vi "Get Moving Status.vi"(8 "error in (no error)":errorcluster, 11 "SIM Motion Controller in":refnum<class "Fine SIM Motion Controller.lvclass">) -> (0 "error out":errorcluster, 2 "Axis Parameters.Moving":bool, 3 "SIM Motion Controller out":refnum<class "Fine SIM Motion Controller.lvclass">)   [LabVIEW 2022 SP3, in "Fine SIM Motion Controller.lvclass"]
uses:
  Fine SIM Motion Controller.lvclass
  C:/Stage-Work/MAS/Axis Objects/Motion Controller/Parent SIM Motion Controller.lvclass
  Motion Controller/Parent SIM Motion Controller.lvclass/Parent SIM Motion Controller.ctl
  Motion Controller/Accessors/Read Sim Axis Data.vi
  Motion Controller/Accessors/Write Sim Axis Data.vi
  Fine SIM Motion Controller.lvclass/Fine SIM Motion Controller.ctl
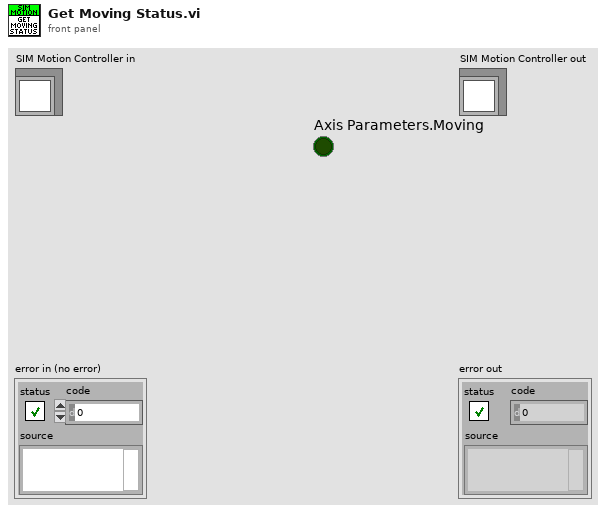
[diagram p1: front panel]
types:
  T1 = typedef "Parent SIM Motion Controller.lvclass/Axis Data.ctl" = cluster{"Axis Parameters":T2, "Axis Settings":T3, "Time Stamp":timestamp}
  T2 = typedef "Parent SIM Motion Controller.lvclass/Axis Parameters.ctl" = cluster{"Moving":bool, "Homed":bool, "Desired Position":dbl, "Current Positon":dbl, "Current Speed":dbl}
  T3 = typedef "Parent SIM Motion Controller.lvclass/Axis Settings.ctl" = cluster{"Speed":dbl, "Acceleration":dbl}
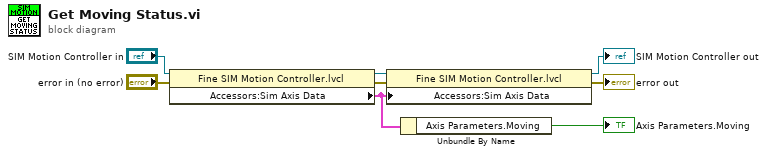
[diagram p0: block diagram]
diagram:
  n1 = property class="Fine SIM Motion Controller.lvcl"(reference="SIM Motion Controller in", error in="error in (no error)") -> (reference out=w6:refnum<class "Fine SIM Motion Controller.lvclass">, error out=w4:errorcluster, "Accessors:Sim Axis Data"=w1:T1)
  n2 = property class="Fine SIM Motion Controller.lvcl"(reference=w6, error in=w4, "Accessors:Sim Axis Data"=w1) -> (reference out=→"SIM Motion Controller out":refnum<class "Fine SIM Motion Controller.lvclass">, error out=→"error out":errorcluster)
  n3 = Unbundle By Name(w1) -> ("Axis Parameters.Moving"=→"Axis Parameters.Moving":bool)
